vi "GetDLLPaths.vi"() -> (0 "etc_xcite_path":path, 1 "PCO_Conv_Path":path, 2 "PCO_Recorder_Path":path, 3 "SC2_Cam_Path":path)   [LabVIEW 2019]
doc: "Returns the absolut paths of the pco DLLs according to the LabVIEW Bitness\nSC2_Cam.dll\nPCO_Recorder.dll\nPCO_Conv.dll"
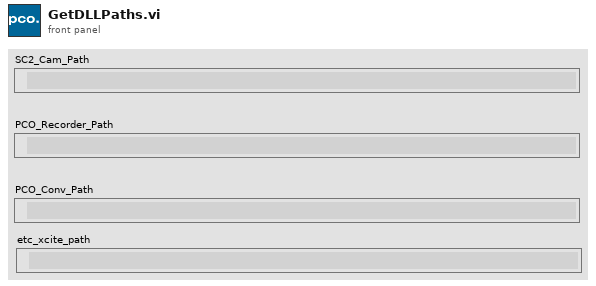
[diagram p1: front panel]
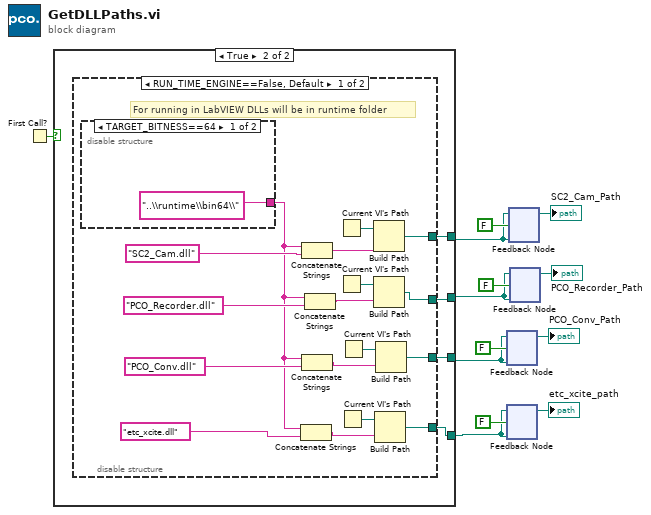
[diagram p0: block diagram]
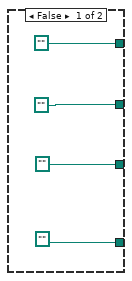
[diagram p2: hidden frame]
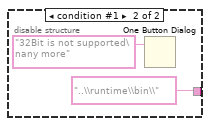
[diagram p3: hidden frame]
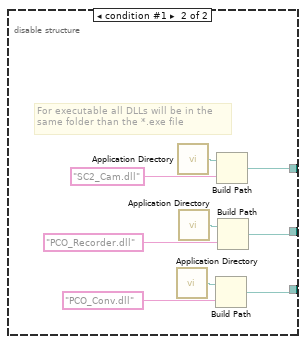
[diagram p4: hidden frame]
diagram:
  n1 = First Call?() -> (First Call?: T/F=w10:bool)
  n2 = case shown="True" w10 {
    tunnel: [path "" w21] -> w11
    tunnel: [path "" w20] -> w4
    tunnel: [path "" w19] -> w5
    tunnel: [path "" w18] -> w1
    frame False {
    }
    frame True {
      n3 = disable-structure shown="RUN_TIME_ENGINE==False, Default" {
        disable-tunnel: [w29 w48] -> w21
        disable-tunnel: [w28 w45] -> w20
        disable-tunnel: [w27 w44] -> w19
        disable-tunnel: [w24 _] -> w18
        frame condition #0 (active) {
          # "For running in LabVIEW DLLs will be in runtime folder"
          n4 = disable-structure shown="TARGET_BITNESS==64" {
            disable-tunnel: ["..\\runtime\\bin64\\" "..\\runtime\\bin\\"] -> w23
            frame condition #0 (active) {
            }
            frame condition #1 {
              n5 = One Button Dialog(message="32Bit is not supported\nany more") -> ()  [unwired: 1 in, 1 out]
            }
          }
          n6 = Concatenate Strings(w23, "etc_xcite.dll") -> (w26:string)
          n7 = Concatenate Strings(w23, "SC2_Cam.dll") -> (w36:string)
          n8 = Concatenate Strings(w23, "PCO_Conv.dll") -> (w31:string)
          n9 = Concatenate Strings(w23, "PCO_Recorder.dll") -> (w30:string)
          n10 = Current VI's Path() -> (path=w38:path)
          n11 = Current VI's Path() -> (path=w33:path)
          n12 = Current VI's Path() -> (path=w25:path)
          n13 = Current VI's Path() -> (path=w32:path)
          n14 = Build Path(base path=w38, name or relative path=w36) -> (appended path=w29:path)
          n15 = Build Path(base path=w33, name or relative path=w30) -> (appended path=w28:path)
          n16 = Build Path(base path=w25, name or relative path=w26) -> (appended path=w24:path)
          n17 = Build Path(base path=w32, name or relative path=w31) -> (appended path=w27:path)
        }
        frame condition #1 {
          # "For executable all DLLs will be in the \nsame folder than the *.exe file"
          n18 = call <vilib>:"Application Directory.vi"() -> ("Application Directory"=w46:path)
          n19 = call <vilib>:"Application Directory.vi"() -> ("Application Directory"=w50:path)
          n20 = call <vilib>:"Application Directory.vi"() -> ("Application Directory"=w47:path)
          n21 = Build Path(base path=w46, name or relative path="PCO_Conv.dll") -> (appended path=w44:path)
          n22 = Build Path(base path=w50, name or relative path="SC2_Cam.dll") -> (appended path=w48:path)
          n23 = Build Path(base path=w47, name or relative path="PCO_Recorder.dll") -> (appended path=w45:path)
        }
      }
    }
  }
  n24 = feedback #1(w5) -> (→"PCO_Conv_Path":path)
  n25 = feedback-in #1(w5, FALSE) -> ()
  n26 = feedback #2(w1) -> (→"etc_xcite_path":path)
  n27 = feedback-in #2(w1, FALSE) -> ()
  n28 = feedback #3(w11) -> (→"SC2_Cam_Path":path)
  n29 = feedback-in #3(w11, FALSE) -> ()
  n30 = feedback #4(w4) -> (→"PCO_Recorder_Path":path)
  n31 = feedback-in #4(w4, FALSE) -> ()
